vi "_write.vi"(8 "Error in (no error)":errorcluster, 10 "Log in":T1 {"Priority" items=["EMERGENCY", "ALERT", "CRITICAL", "ERROR", "WARNING", "NOTICE", "INFO", "DEBUG"]}, 11 "LogWriterInterface in":refnum<class "LogWriterInterface.lvclass">) -> (0 "Error out":errorcluster, 3 "LogWriterInterface out":refnum<class "LogWriterInterface.lvclass">)   [LabVIEW 2011, in "LogWriterInterface.lvclass"]
uses:
  LogWriterInterface.lvclass
  Log/LogCluster.ctl
  Log/PrioritiesRing.ctl
  Log/Log.lvclass
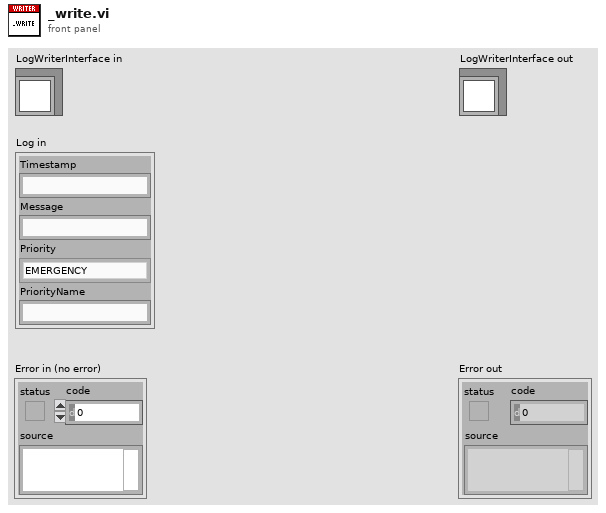
[diagram p1: front panel]
types:
  T1 = typedef "Log.lvclass/LogCluster.ctl" = cluster{"Timestamp":string, "Message":string, "Priority":T2, "PriorityName":string}
  T2 = typedef "Log.lvclass/PrioritiesRing.ctl" = u32
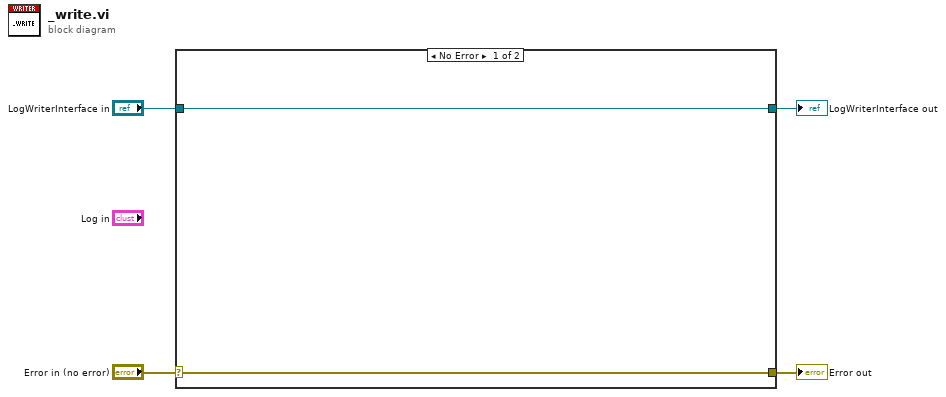
[diagram p0: block diagram]
diagram:
  n1 = case shown="No Error" "Error in (no error)" {
    selector: "Error in (no error)" -> [w5 w8]
    tunnel: [w5 w8] -> w3
    tunnel: [w6 w7] -> w1
    tunnel: "LogWriterInterface in" -> [w6 w7]
    frame No Error {
    }
    frame Error {
    }
  }
  "Error out" <- w3
  "LogWriterInterface out" <- w1
